vi "updateTasksToList.vi"(8 "error in (no error)":errorcluster, 10 "Selected Tasks":refnum<class "Task.lvclass">[](array[class]), 11 "BuildServer in":refnum<class "BuildServer.lvclass">) -> (0 "error out":errorcluster)   [LabVIEW 2017, in "BuildServer.lvlib" / "BuildServer.lvclass"]
uses:
  BuildServer.lvclass
  <vilib>/Ekim/LUT/LUT/LUT.lvclass
  BuildWorker/Classes/Task/Task.lvclass
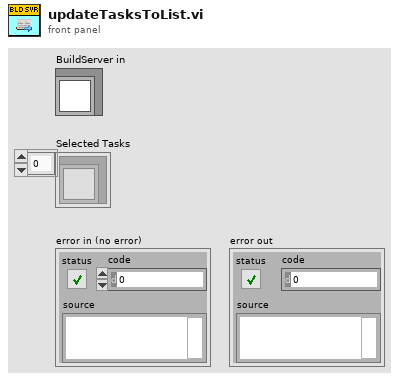
[diagram p1: front panel]
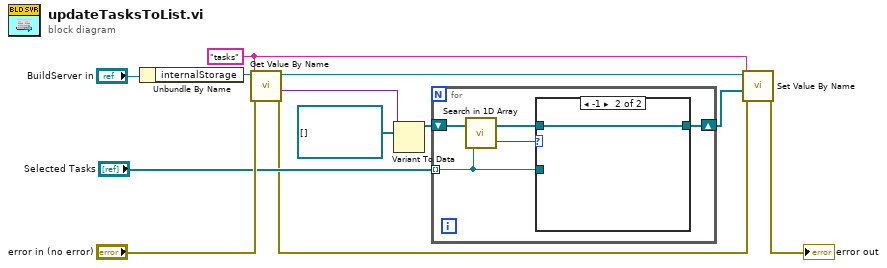
[diagram p0: block diagram]
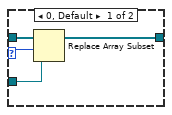
[diagram p2: hidden frame]
diagram:
  w10 = "tasks" ("Name")
  n1 = Unbundle By Name("BuildServer in") -> ("internalStorage"=w3:refnum<class "LUT.lvclass">)
  n2 = call <vilib>:"Get Value By Name.vi"("error in (no error)"="error in (no error)", "Name"=w10, "LUT in"=w3) -> ("error out"=w1:errorcluster, "Value"=w4:variant, "LUT out"=w8:refnum<class "LUT.lvclass">)  [unwired: 5 in, 1 out]
  n3 = Variant To Data(type=refnum<class "Task.lvclass">[] [] ("Selected Tasks"), Variant=w4) -> (data=w6:refnum<class "Task.lvclass">[])  [unwired: 1 in, 1 out]
  n4 = for {
    tunnel: "Selected Tasks" -> [w14] mode=indexing
    shift-right: [w16] -> w9
    shift-left: w6 -> [w13]
    n5 = call "Search in 1D Array.vi"("Task in"=w14, "Task Array"=w13) -> ("index of element"=w15:i32)  [unwired: 1 out]
    n6 = case shown="-1" w15 {
      selector: w15 -> [w19 _]
      tunnel: [w20 w21] -> w16
      tunnel: w14 -> [w18 _]
      tunnel: w13 -> [w17 w21]
      frame 0, Default {
        n7 = Replace Array Subset(array=w17, new element=w18, index=w19) -> (w20:refnum<class "Task.lvclass">[])
      }
      frame -1 {
      }
    }
  }
  n8 = call <vilib>:"Set Value By Name.vi"("error in (no error)"=w1, "Value"=w9, "Name"=w10, "LUT in"=w8) -> ("error out"=→"error out":errorcluster)  [unwired: 5 in, 2 out]
